vi "Draw.vi"(8 "error in (no error)":errorcluster, 10 "2D Picture in":picture, 11 "Collection in":refnum<class "Collection.lvclass">) -> (0 "error out":errorcluster, 2 "2D Picture out":picture, 3 "Collection out":refnum<class "Collection.lvclass">)   [LabVIEW 2021, in "Picture2D.lvlib" / "Collection.lvclass"]
uses:
  Collection.lvclass
  Collection.lvclass/Collection.ctl
  IDrawable/IDrawable.lvclass
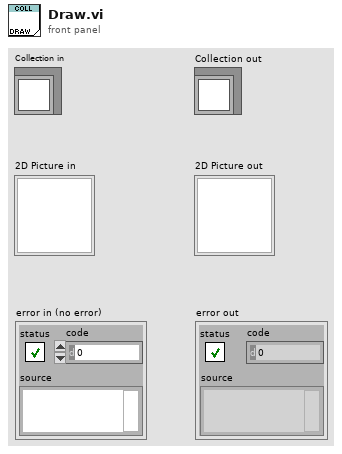
[diagram p1: front panel]
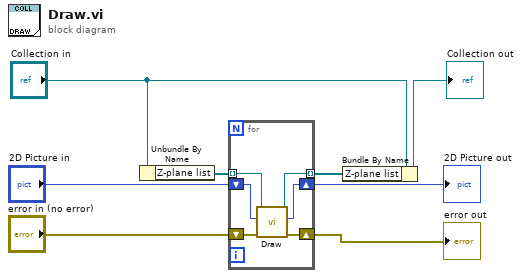
[diagram p0: block diagram]
diagram:
  n1 = Unbundle By Name("Collection in") -> ("Z-plane list"=w7:refnum<class "IDrawable.lvclass">[])
  n2 = for {
    shift-right: [w12] -> w5
    shift-left: "2D Picture in" -> [w11]
    tunnel: w7 -> [w14] mode=indexing
    tunnel: [w13] -> w6 mode=indexing
    shift-right: [w9] -> w1
    shift-left: "error in (no error)" -> [w10]
    n3 = call-dynamic "Draw.vi"("error in (no error)"=w10, "2D Picture in"=w11, "IDrawable in"=w14) -> ("error out"=w9:errorcluster, "2D Picture out"=w12:picture, "IDrawable out"=w13:refnum<class "IDrawable.lvclass">)  [unwired: 6 in]
  }
  "error out" <- w1
  "2D Picture out" <- w5
  n4 = Bundle By Name(cluster="Collection in", "Z-plane list"=w6) -> (→"Collection out":refnum<class "Collection.lvclass">)
